vi "Scan Engine Convert Module String.vi"(1 "Module Name":string) -> (0 "Module":T1)   [LabVIEW 2016, in "Scan Engine Custom Device.lvlib"]
uses:
  Scan Engine Custom Device.lvlib
  Modules.lvlibp/RSI Module/Module Models.ctl
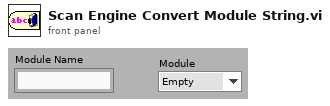
[diagram p1: front panel]
types:
  T1 = typedef "Modules.lvlibp/RSI Module.lvclass/Module Models.ctl" = enum16{"Empty", "NI 9201", "NI 9203", "NI 9205", "NI 9206", "NI 9207", "NI 9208", "NI 9211", "NI 9213", "NI 9214", "NI 9215", "NI 9217", "NI 9219", "NI 9221", "NI 9225", "NI 9227", "NI 9229", "NI 9233", "NI 9234", "NI 9235", "NI 9236", "NI 9237", "NI 9239", "NI 9263", "NI 9264", "NI 9265", "NI 9269", "NI 9375", "NI 9401", "NI 9402", "NI 9403", "NI 9411", "NI 9421", "NI 9422", "NI 9423", "NI 9425", "NI 9426", "NI 9435", "NI 9472", "NI 9474", "NI 9475", "NI 9476", "NI 9477", "NI 9478", "NI 9481", "NI 9482", "NI 9485"}
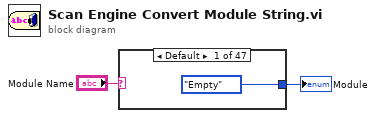
[diagram p0: block diagram]
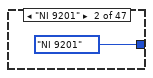
[diagram p2: hidden frame]
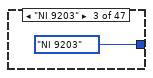
[diagram p3: hidden frame]
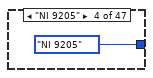
[diagram p4: hidden frame]
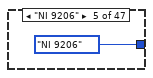
[diagram p5: hidden frame]
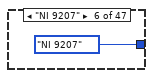
[diagram p6: hidden frame]
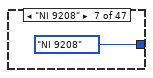
[diagram p7: hidden frame]
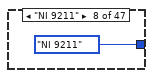
[diagram p8: hidden frame]
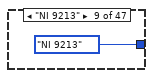
[diagram p9: hidden frame]
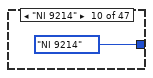
[diagram p10: hidden frame]
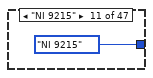
[diagram p11: hidden frame]
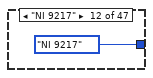
[diagram p12: hidden frame]
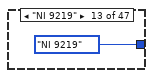
[diagram p13: hidden frame]
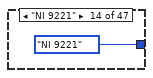
[diagram p14: hidden frame]
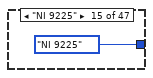
[diagram p15: hidden frame]
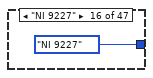
[diagram p16: hidden frame]
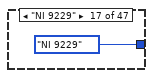
[diagram p17: hidden frame]
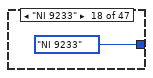
[diagram p18: hidden frame]
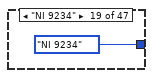
[diagram p19: hidden frame]
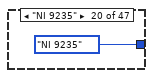
[diagram p20: hidden frame]
diagram:
  n1 = case shown="Default" "Module Name" {
    tunnel: [Module_Models."Empty" ("Module") Module_Models."NI 9201" ("Module") Module_Models."NI 9203" ("Module") Module_Models."NI 9205" ("Module") Module_Models."NI 9206" ("Module") Module_Models."NI 9207" ("Module") Module_Models."NI 9208" ("Module") Module_Models."NI 9211" ("Module") Module_Models."NI 9213" ("Module") Module_Models."NI 9214" ("Module") Module_Models."NI 9215" ("Module") Module_Models."NI 9217" ("Module") Module_Models."NI 9219" ("Module") Module_Models."NI 9221" ("Module") Module_Models."NI 9225" ("Module") Module_Models."NI 9227" ("Module") Module_Models."NI 9229" ("Module") Module_Models."NI 9233" ("Module") Module_Models."NI 9234" ("Module") Module_Models."NI 9235" ("Module") Module_Models."NI 9236" ("Module") Module_Models."NI 9237" ("Module") Module_Models."NI 9239" ("Module") Module_Models."NI 9263" ("Module") Module_Models."NI 9264" ("Module") Module_Models."NI 9265" ("Module") Module_Models."NI 9269" ("Module") Module_Models."NI 9375" ("Module") Module_Models."NI 9401" ("Module") Module_Models."NI 9402" ("Module") Module_Models."NI 9403" ("Module") Module_Models."NI 9411" ("Module") Module_Models."NI 9421" ("Module") Module_Models."NI 9422" ("Module") Module_Models."NI 9423" ("Module") Module_Models."NI 9425" ("Module") Module_Models."NI 9426" ("Module") Module_Models."NI 9435" ("Module") Module_Models."NI 9472" ("Module") Module_Models."NI 9474" ("Module") Module_Models."NI 9475" ("Module") Module_Models."NI 9476" ("Module") Module_Models."NI 9477" ("Module") Module_Models."NI 9478" ("Module") Module_Models."NI 9481" ("Module") Module_Models."NI 9482" ("Module") Module_Models."NI 9485" ("Module")] -> w1
    frame Default {
    }
    frame "NI 9201" {
    }
    frame "NI 9203" {
    }
    frame "NI 9205" {
    }
    frame "NI 9206" {
    }
    frame "NI 9207" {
    }
    frame "NI 9208" {
    }
    frame "NI 9211" {
    }
    frame "NI 9213" {
    }
    frame "NI 9214" {
    }
    frame "NI 9215" {
    }
    frame "NI 9217" {
    }
    frame "NI 9219" {
    }
    frame "NI 9221" {
    }
    frame "NI 9225" {
    }
    frame "NI 9227" {
    }
    frame "NI 9229" {
    }
    frame "NI 9233" {
    }
    frame "NI 9234" {
    }
    frame "NI 9235" {
    }
    frame "NI 9236" {
    }
    frame "NI 9237" {
    }
    frame "NI 9239" {
    }
    frame "NI 9263" {
    }
    frame "NI 9264" {
    }
    frame "NI 9265" {
    }
    frame "NI 9269" {
    }
    frame "NI 9375" {
    }
    frame "NI 9401" {
    }
    frame "NI 9402" {
    }
    frame "NI 9403" {
    }
    frame "NI 9411" {
    }
    frame "NI 9421" {
    }
    frame "NI 9422" {
    }
    frame "NI 9423" {
    }
    frame "NI 9425" {
    }
    frame "NI 9426" {
    }
    frame "NI 9435" {
    }
    frame "NI 9472" {
    }
    frame "NI 9474" {
    }
    frame "NI 9475" {
    }
    frame "NI 9476" {
    }
    frame "NI 9477" {
    }
    frame "NI 9478" {
    }
    frame "NI 9481" {
    }
    frame "NI 9482" {
    }
    frame "NI 9485" {
    }
  }
  "Module" <- w1
